vi "Parse Core.vi"(0 "Path in":refnum<class "Path.lvclass">, 5 "Config Row":string[](array[string]), 11 "error in (no error)":errorcluster) -> (4 "Path out":refnum<class "Path.lvclass">, 15 "error out":errorcluster)   [LabVIEW 2023, in "RFCalAndFixtureCharact.Common.lvlib" / "Path.lvclass"]
uses:
  Path.lvclass
  Path.lvclass/Path.ctl
  Properties/Write Interval.vi
  Properties/Write Date.vi
  RFCalAndFixtureCharact.Common.lvlib
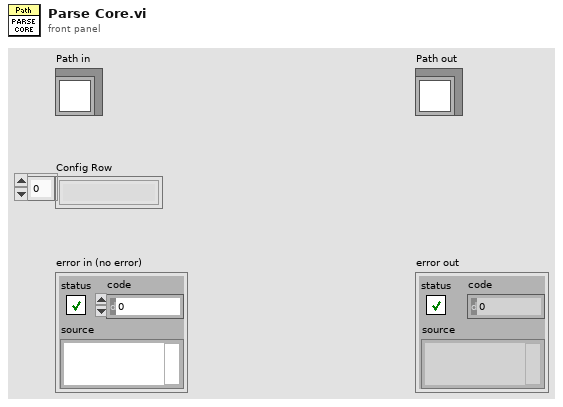
[diagram p1: front panel]
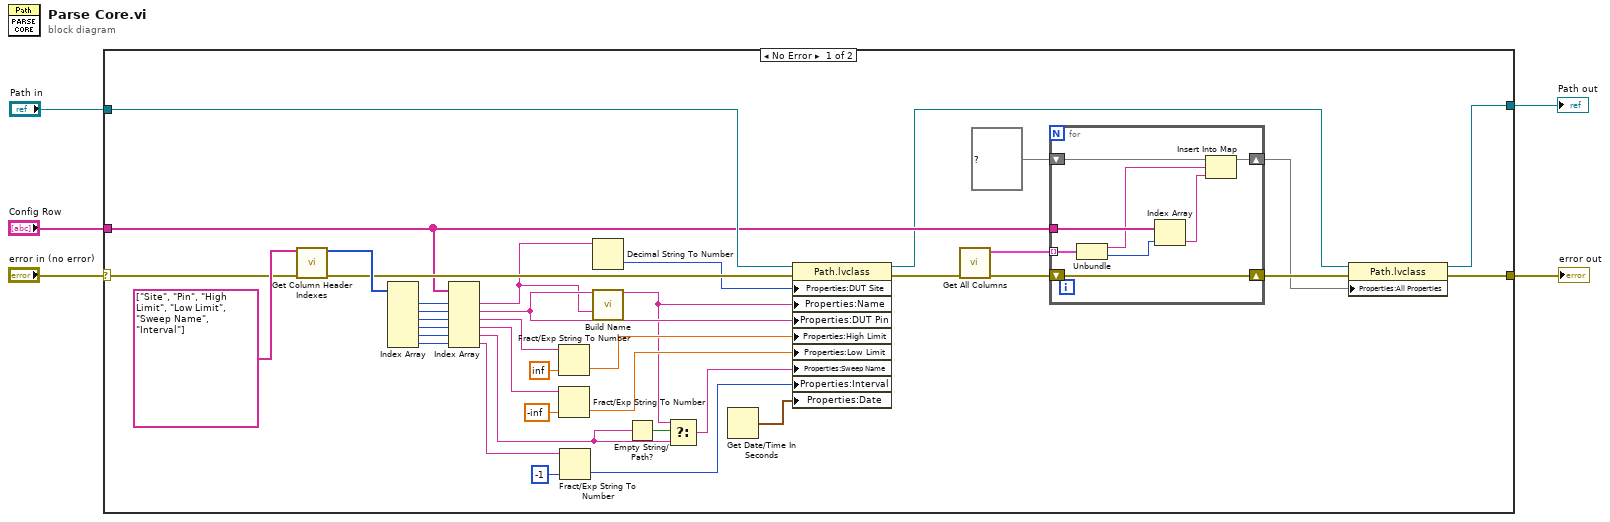
[diagram p0: block diagram]
diagram:
  n1 = case shown="No Error" "error in (no error)" {
    selector: "error in (no error)" -> [w36 w53]
    tunnel: [w10 w53] -> w4
    tunnel: [w7 w52] -> w2
    tunnel: "Path in" -> [w38 w52]
    tunnel: "Config Row" -> [w11 _]
    frame No Error {
      n2 = call "Get Column Header Indexes.vi"("Column Header Names"=string[] ["Site", "Pin", "High Limit", "Low Limit", "Sweep Name", "Interval"], "error in"=w36) -> ("Column Header Indices"=w35:i32[], "error out"=w29:errorcluster)  [unwired: 11 in, 1 out]
      n3 = Index Array(array=w35) -> (element #1=w34:i32, element #2=w33:i32, element #3=w32:i32, element #4=w31:i32, element #5=w30:i32, element #6=w21:i32)  [unwired: 6 in]
      n4 = Index Array(array=w11, index #1=w34, index #2=w33, index #3=w32, index #4=w31, index #5=w30, index #6=w21) -> (element #1=w16:string, element #2=w39:string, element #3=w41:string, element #4=w40:string, element #5=w22:string, element #6=w20:string)
      n5 = Fract/Exp String To Number(string=w41, default (0 dbl)=inf ("default (0 DBL)")) -> (number=w43:dbl)  [unwired: 2 in, 1 out]
      n6 = Fract/Exp String To Number(string=w40, default (0 dbl)=-inf ("default (0 DBL)")) -> (number=w42:dbl)  [unwired: 2 in, 1 out]
      n7 = Fract/Exp String To Number(string=w20, default (0 dbl)=-1 ("Interval")) -> (number=w18:i32)  [unwired: 2 in, 1 out]
      n8 = Decimal String To Number(string=w16) -> (number=w26:i32)  [unwired: 2 in, 1 out]
      n9 = call "Build Name.vi"("Pin"=w39, "Site"=w16) -> ("Path name"=w23:string)  [unwired: 13 in]
      n10 = Empty String/Path?(string/path=w22) -> (empty?=w25:bool)
      n11 = Select(t=w23, s=w25, f=w22) -> (s? t:f=w24:string)
      n12 = Get Date/Time In Seconds() -> (seconds since 1Jan1904=w17:timestamp)
      n13 = property class="Path.lvclass"(reference=w38, error in=w29, "Properties:DUT Site"=w26, "Properties:Name"=w23, "Properties:DUT Pin"=w39, "Properties:High Limit"=w43, "Properties:Low Limit"=w42, "Properties:Sweep Name"=w24, "Properties:Interval"=w18, "Properties:Date"=w17) -> (reference out=w9:refnum<class "Path.lvclass">, error out=w13:errorcluster)
      n14 = call "Get All Columns.vi"("error in (no error)"=w13) -> ("All Columns out"=w6:cluster{string, i32}[], "error out"=w14:errorcluster)  [unwired: 13 in]
      n15 = for {
        tunnel: w11 -> [w51]
        shift-right: [w49] -> w8
        shift-left: map{string, string} {} ("Custom Columns") -> [w48]
        shift-right: [w47] -> w12
        shift-left: w14 -> [w47]
        tunnel: w6 -> [w46] mode=indexing
        n16 = Unbundle(w46) -> (w45:string, w44:i32)
        n17 = Index Array(array=w51, index=w44) -> (element=w50:string)
        n18 = Insert Into Map(map in=w48, key=w45, value=w50) -> (map out=w49:map{string, string})  [unwired: 2 out]
      }
      n19 = property class="Path.lvclass"(reference=w9, error in=w12, "Properties:All Properties"=w8) -> (reference out=w7:refnum<class "Path.lvclass">, error out=w10:errorcluster)
    }
    frame Error {
    }
  }
  "error out" <- w4
  "Path out" <- w2
